vi "TurnCrank.vi"(8 "error in (no error)":errorcluster, 11 "object in":refnum<class "SoldState.lvclass">) -> (0 "error out":errorcluster, 3 "object out":refnum<class "State.lvclass">)   [LabVIEW 2020, in "SoldState.lvclass"]
uses:
  SoldState.lvclass
  C:/Projects/OpenGDS_DesignPatterns/State1/State_class/State.lvclass
  State_class/State.lvclass
  SoldState.lvclass/SoldState.ctl
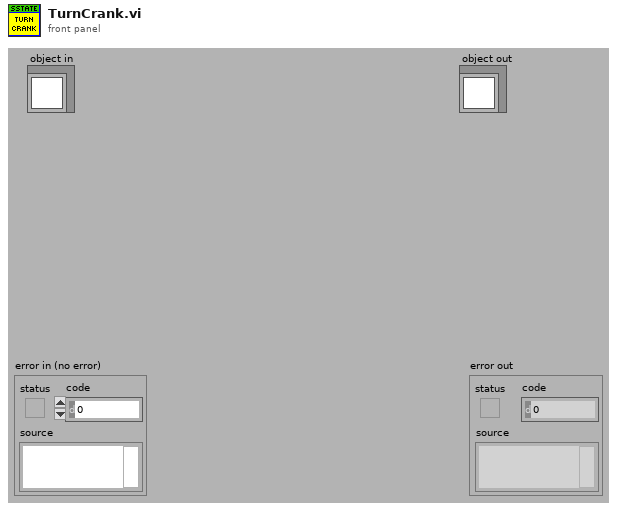
[diagram p1: front panel]
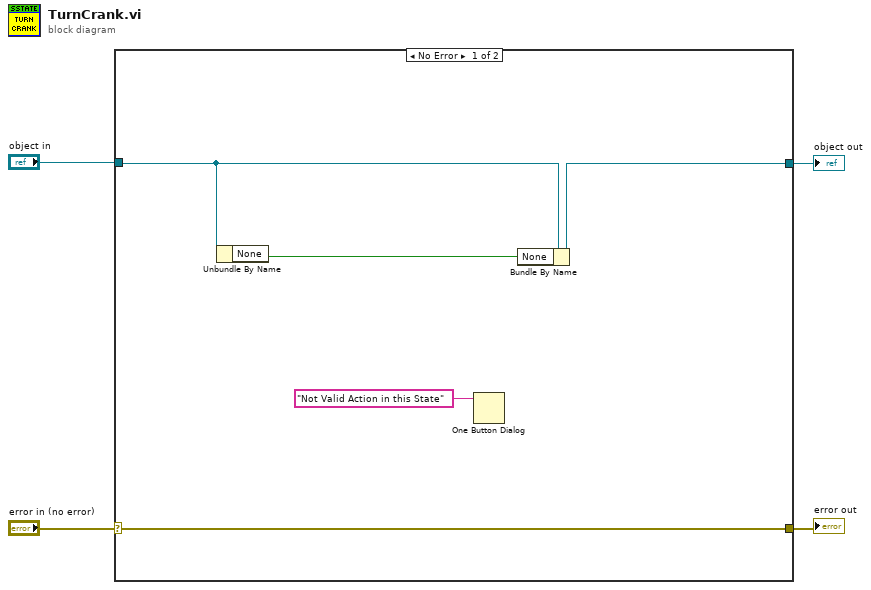
[diagram p0: block diagram]
diagram:
  n1 = case shown="No Error" "error in (no error)" {
    selector: "error in (no error)" -> [w8 w11]
    tunnel: [w8 w11] -> w3
    tunnel: [w6 w10] -> w1
    tunnel: "object in" -> [w7 w10]
    frame No Error {
      n2 = Unbundle By Name(w7) -> ("None"=w9:bool)
      n3 = One Button Dialog(message="Not Valid Action in this State" ("TextIn")) -> ()  [unwired: 1 in, 1 out]
      n4 = Bundle By Name(cluster=w7, "None"=w9) -> (w6:refnum<class "SoldState.lvclass">)
    }
    frame Error {
    }
  }
  "error out" <- w3
  "object out" <- w1
